vi "Align Waveforms by Leading Sync Pulse.vi"(6 "maximum delay":i32=51200, 7 "reset":bool, 8 "error in (no error)":errorcluster, 9 "tolerance":dbl=0.1 format="%#_13g", 10 "response signals":waveform(dbl)[](array[waveform]), 11 "alignment reference signal":waveform(dbl)={"t0"=timestamp(0 s since 1904-01-01), "dt"=0.0, "Y"=[]}) -> (0 "error out":errorcluster, 1 "residual delays [s]":dbl[](array[numeric]) format="%.2p", 2 "aligned signals":waveform(dbl)[](array[waveform]), 4 "aligned signals length":i32, 5 "alignment reference detected":bool)   [LabVIEW 2022 SP3]
doc: "Use this VI to measure the delay from reference to each response and effectively remove the integer sample delay on each channel in order to align the responses according to expected reference signal."
uses:
  <vilib>/addons/Sound and Vibration/svt_Calibration/SV Measure Delay and Polarity and Coherence (Nx1).vi
  Program Files/NI/LVAddons/nisvt/1/examples/Sound and Vibration/Audio Measurements/subVIs/sv_Assign Delay to Idle Channels.vi
  <vilib>/addons/_NISVFA/_Shared subVIs/Common/svc_Check for Waveform Parameter Continuity (N Ch).vi
  <vilib>/addons/Sound and Vibration/svt_Calibration/SV Measure Delay and Polarity and Coherence.vi
  <vilib>/addons/_NISVFA/_Shared subVIs/Common/sv_Get NI Property Name String.vi
  <vilib>/addons/_NISVFA/_Shared subVIs/Common/svc_Check for Waveform Parameter Continuity (no state).vi
  <vilib>/Analysis/_algsub.llb/Vector Norm.vi
  <vilib>/Analysis/_algsub.llb/Real Vector Norm.vi
  <vilib>/addons/_NISVFA/_Shared subVIs/Common/SV Get Data Subset.vi
  <vilib>/addons/_NISVFA/_Shared subVIs/Common/svc_Get Array Subset (Index).vi
  <vilib>/addons/_NISVFA/_Shared subVIs/Common/svc_Get SV Channel Info.vi
  <vilib>/addons/_NISVFA/_Shared subVIs/Common/svc_Coerce Index and Length.vi
  <vilib>/addons/_NISVFA/_Shared subVIs/Common/svc_Unit Label to Engineering Units.vi
  <vilib>/addons/_NISVFA/_Shared subVIs/Common/svc_Engineering Units to Unit Label.vi
  <vilib>/addons/_NISVFA/_Shared subVIs/Common/svc_Conditional Merge Error.vi
  <vilib>/addons/_NISVFA/_Shared subVIs/Data Objects/Waveforms (DBL)/SV Read Newest Data.vi
  <vilib>/measure/maresamp.llb/Resample Waveforms (single shot).vi
  <vilib>/measure/maresamp.llb/Resample Waveform (single shot).vi
  <vilib>/addons/_NISVFA/_Shared subVIs/Common/svc_Check dt for Equal Sample Rates.vi
  <vilib>/Waveform/TSOps.llb/Timestamp Subtract.vi
  <vilib>/Analysis/2dsp.llb/CrossCorrelation.vi
  <vilib>/Analysis/2dsp.llb/1D Cross Correlation (DBL).vi
  <vilib>/addons/_NISVFA/_Shared subVIs/Common/svc_Fit Quadratic to Max Three Points in Array.vi
  <vilib>/Utility/error.llb/Error Cluster From Error Code.vi
  <vilib>/addons/_NISVFA/_Shared subVIs/Common/svc_Caller VI Returned in Error Source.vi
  <vilib>/addons/_NISVFA/_Shared subVIs/Data Objects/Waveforms (DBL)/Waveforms (N Ch).lvclass
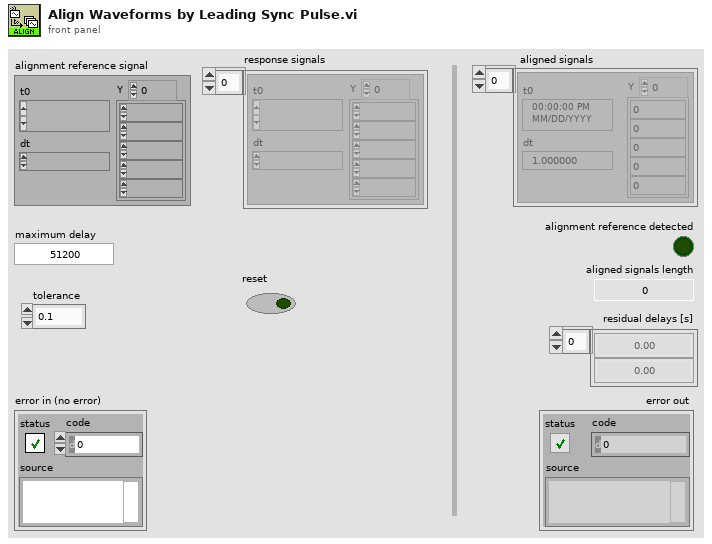
[diagram p1: front panel]
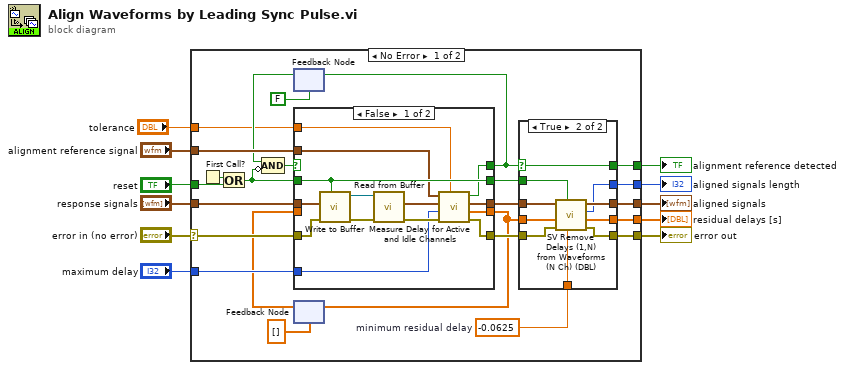
[diagram p0: block diagram]
diagram:
  n1 = case shown="No Error" "error in (no error)" {
    selector: "error in (no error)" -> [w32 w68]
    tunnel: "response signals" -> [w35 _]
    tunnel: "alignment reference signal" -> [w34 _]
    tunnel: "maximum delay" -> [w33 _]
    tunnel: [w14 _] -> w7
    tunnel: [w27 _] -> w6
    tunnel: [w26 _] -> w5
    tunnel: [w25 _] -> w4
    tunnel: "reset" -> [w19 _]
    tunnel: [w15 w68] -> w2
    tunnel: "tolerance" -> [w12 _]
    frame No Error {
      w13 = -0.0625  # minimum residual delay
      n2 = First Call?() -> (First Call?: T/F=w20:bool)
      n3 = Or(x=w20, y=w19) -> (x .or. y?=w18:bool)
      n4 = feedback #1(FALSE) -> (w17:bool)
      n5 = Compound Arithmetic op=AND(w17, invert w18) -> (w16:bool)
      n6 = feedback #2(dbl[] [] ("Array")) -> (w22:dbl[])
      n7 = case shown="False" w16 {
        selector: w16 -> [_ w53]
        tunnel: w35 -> [w46 w54]
        tunnel: w34 -> [w40 _]
        tunnel: w33 -> [w39 _]
        tunnel: w32 -> [w49 w52]
        tunnel: [w47 w52] -> w31
        tunnel: [w37 w54] -> w30
        tunnel: [w38 w53] -> w29
        tunnel: [w42 w51] -> w23
        tunnel: w22 -> [_ w51]
        tunnel: w18 -> [w48 w50]
        tunnel: [w48 w50] -> w21
        tunnel: w12 -> [w36 _]
        frame False {
          n8 = call <vilib>:"Write to Buffer.vi"("clear buffer (False)"=w48, "error in (no error)"=w49, "waveforms"=w46) -> ("error out"=w44:errorcluster, "buffer out"=w45:refnum<data-value>)  [unwired: 6 in, 1 out]
          n9 = call-poly <vilib>:"Read from Buffer.vi"("error in (no error)"=w44, "buffer"=w45) -> ("error out"=w43:errorcluster, "waveforms subset"=w41:waveform(dbl)[])  [unwired: 6 in, 2 out]
          n10 = call "Measure Delay for Active and Idle Channels.vi"("tolerance"=w36, "error in (no error)"=w43, "maximum delay"=w39, "waveforms subset"=w41, "alignment reference signal"=w40) -> ("error out"=w47:errorcluster, "delays [s]"=w42:dbl[], "waveforms subset dup"=w37:waveform(dbl)[], "reference detected"=w38:bool)  [unwired: 3 in]
        }
        frame True {
        }
      }
      n11 = feedback-in #1(w29) -> ()
      n12 = feedback-in #2(w23) -> ()
      n13 = case shown="True" w29 {
        selector: w29 -> [w56 w59]
        tunnel: w31 -> [w57 w67]
        tunnel: w30 -> [w55 w66]
        tunnel: w21 -> [_ w65]
        tunnel: w23 -> [_ w63]
        tunnel: [w55 w64] -> w27
        tunnel: [_ w62] -> w26
        tunnel: [_ w61] -> w25
        tunnel: [w57 w60] -> w15
        tunnel: [w56 w59] -> w14
        tunnel: w13 -> [_ w58]
        frame False {
        }
        frame True {
          n14 = call <vilib>:"SV Remove Delays (1,N) from Waveforms (N Ch) (DBL).vi"("minimum residual delay"=w58, "reset"=w65, "error in (no error)"=w67, "path-dependent analog delays [s]"=w63, "scaled signals"=w66) -> ("error out"=w60:errorcluster, "residual delays [s]"=w61:dbl[], "aligned signals length"=w62:i32, "aligned signals"=w64:waveform(dbl)[])  [unwired: 3 in]
        }
      }
    }
    frame Error {
    }
  }
  "aligned signals" <- w6
  "alignment reference detected" <- w7
  "aligned signals length" <- w5
  "residual delays [s]" <- w4
  "error out" <- w2
